vi "Setup subWorker - UI Cam 1.vi"(8 "error in":errorcluster, 11 "Container in":refnum<class "Container.lvclass">) -> (0 "error out":errorcluster, 3 "Container out":refnum<class "Container.lvclass">)   [LabVIEW 2023, in "Container.lvclass"]
doc: "<b>Note: Do not change the code in this VI!</b>\nThis VI performs a setup of all the statically-linked subWorkers that belong to the Worker that calls this VI. This VI is created automatically by the 'Create/Add Worker' tool and must be called <b>before</b> any statically linked subWorkers are called."
uses:
  Container.lvclass
  Container.lvclass/Container.ctl
  UI Cam Basler/UI Cam Basler.lvclass
  C:/Program Files (x86)/National Instruments/LabVIEW 2023/vi.lib/addons/_Workers/Library/Classes/Worker/Worker.lvclass
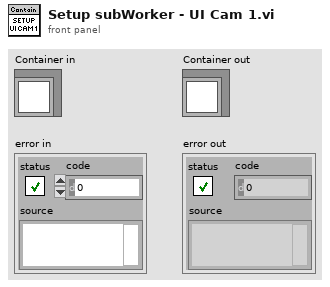
[diagram p1: front panel]
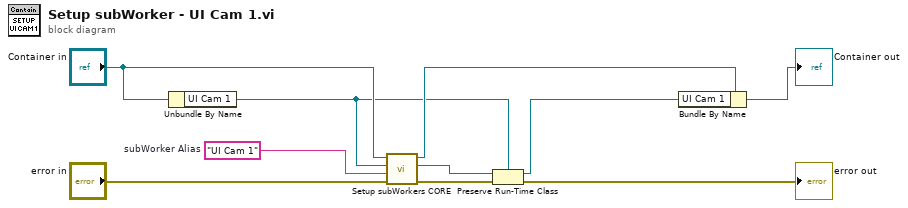
[diagram p0: block diagram]
diagram:
  w6 = "UI Cam 1"  # subWorker Alias
  n1 = Unbundle By Name("Container in") -> ("UI Cam 1"=w3:refnum<class "UI Cam Basler.lvclass">)
  n2 = call-dynamic "Setup subWorkers CORE.vi"("error in"="error in", "subWorker Alias"=w6, "subWorker"=w3, "Worker"="Container in") -> ("error out"=w5:errorcluster, "subWorker out"=w1:refnum<class "Worker.lvclass">, "Worker out"=w8:refnum<class "Container.lvclass">)  [unwired: 5 in]
  n3 = Preserve Run-Time Class(object in=w1, error in=w5, 2:w3) -> (object out=w2:refnum<class "UI Cam Basler.lvclass">, error out=→"error out":errorcluster)
  n4 = Bundle By Name(cluster=w8, "UI Cam 1"=w2) -> (→"Container out":refnum<class "Container.lvclass">)
